vi "PFI-28000-Channel_Create.vi"(0 "PFI-28000-Channel in":refnum<class "PFI-28000-Channel.lvclass">, 5 "Parent":refnum<class "PFI-28000-Card.lvclass">, 7 "Channel Number":i32, 11 "error in (no error)":errorcluster) -> (4 "PFI-28000-Channel out":refnum<class "PFI-28000-Channel.lvclass">, 15 "error out":errorcluster)   [LabVIEW 2017, in "PFI-28000-Channel.lvclass"]
uses:
  PFI-28000-Channel.lvclass
  Card/PFI-28000-Card.lvclass
  C:/wc/07143 Precision Filters 28000 Support/Driver/source/Base/PFI-28000-Base.lvclass
  PFI-28000-Channel.lvclass/PFI-28000-Channel.ctl
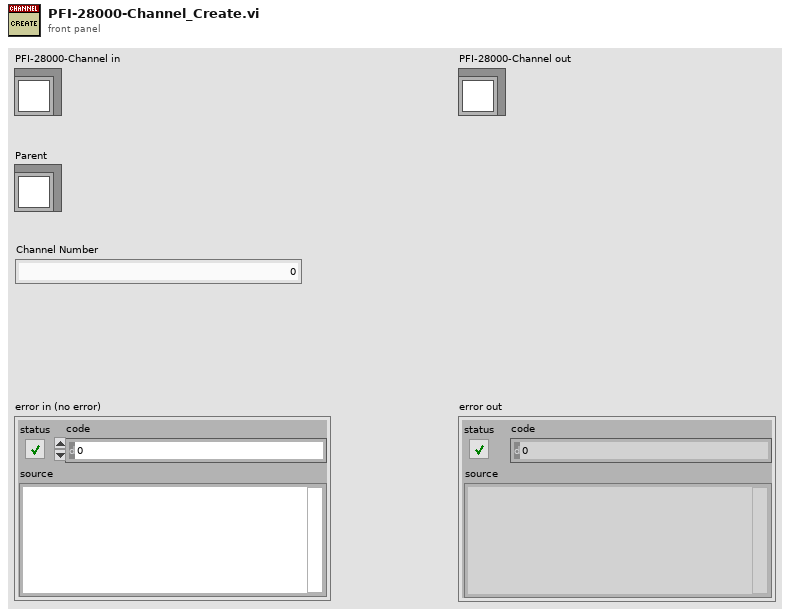
[diagram p1: front panel]
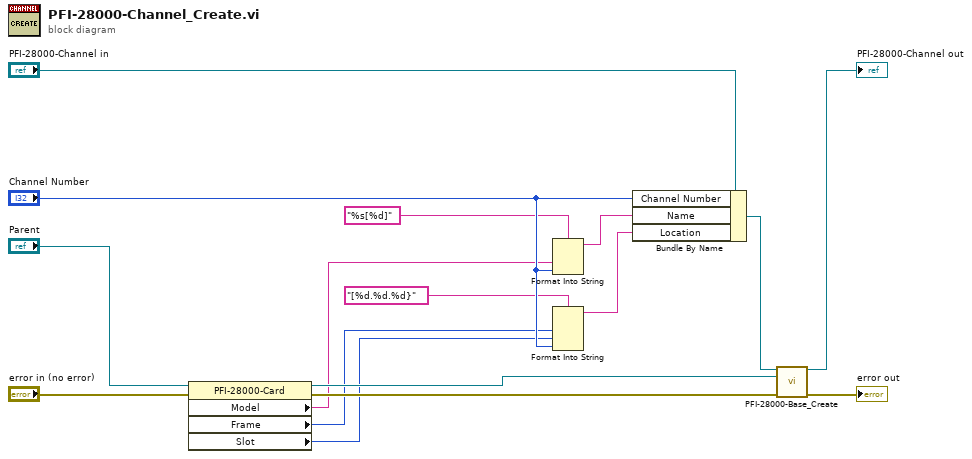
[diagram p0: block diagram]
diagram:
  n1 = property class="PFI-28000-Card"(reference="Parent", error in="error in (no error)") -> (reference out=w15:refnum<class "PFI-28000-Card.lvclass">, error out=w12:errorcluster, "Model"=w6:string, "Frame"=w9:i32, "Slot"=w8:i32)
  n2 = Format Into String(format string="%s[%d]" ("empty string"), w6, "Channel Number") -> (resulting string=w3:string)  [unwired: 2 in, 1 out]
  n3 = Format Into String(format string="[%d.%d.%d}" ("empty string"), w9, w8, "Channel Number") -> (resulting string=w4:string)  [unwired: 2 in, 1 out]
  n4 = Bundle By Name(cluster="PFI-28000-Channel in", "Channel Number"="Channel Number", "Name"=w3, "Location"=w4) -> (w5:refnum<class "PFI-28000-Channel.lvclass">)
  n5 = call-dynamic "PFI-28000-Base_Create.vi"("PFI-28000-Base in"=w5, "Parent"=w15, "error in (no error)"=w12) -> ("PFI-28000-Base out"=→"PFI-28000-Channel out":refnum<class "PFI-28000-Channel.lvclass">, "error out"=→"error out":errorcluster)  [unwired: 11 in]
